vi "Write Timeout (ms).vi"(8 "error in (no error)":errorcluster, 10 "Timeout (ms)":i32=1000, 11 "PIOD in":refnum<class "PIOD.lvclass">) -> (0 "error out":errorcluster, 3 "PIOD out":refnum<class "PIOD.lvclass">)   [LabVIEW 2018, in "PIOD.lvlib" / "PIOD.lvclass"]
uses:
  PIOD.lvclass
  PIOD.lvclass/PIOD.ctl
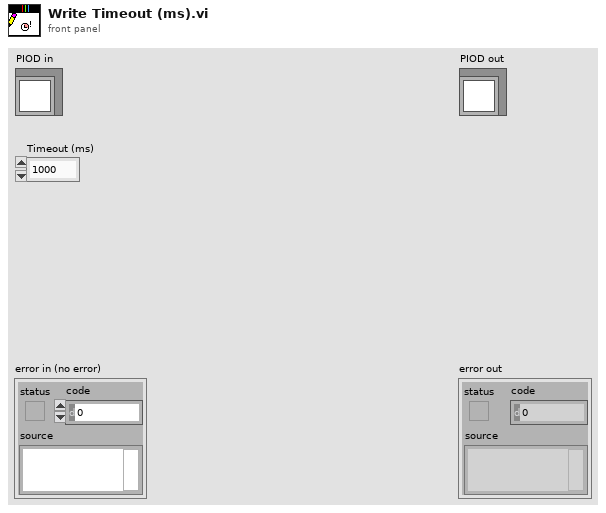
[diagram p1: front panel]
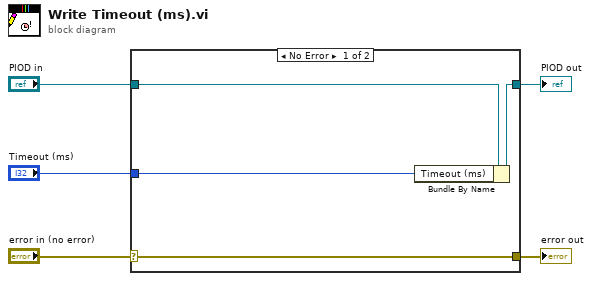
[diagram p0: block diagram]
diagram:
  n1 = case shown="No Error" "error in (no error)" {
    selector: "error in (no error)" -> [w9 w10]
    tunnel: [w9 w10] -> w4
    tunnel: [w7 w11] -> w2
    tunnel: "PIOD in" -> [w8 w11]
    tunnel: "Timeout (ms)" -> [w6 _]
    frame No Error {
      n2 = Bundle By Name(cluster=w8, "Timeout (ms)"=w6) -> (w7:refnum<class "PIOD.lvclass">)
    }
    frame Error {
    }
  }
  "error out" <- w4
  "PIOD out" <- w2
